vi "Read Name.vi"(8 "error in (no error)":errorcluster, 11 "bt_Send_Queue in":refnum<class "bt_Send_Queue.lvclass">) -> (0 "error out":errorcluster, 2 "Name":string, 3 "bt_Send_Queue out":refnum<class "bt_Send_Queue.lvclass">)   [LabVIEW 2021, in "BT.lvlib" / "bt_Send_Queue.lvclass"]
uses:
  bt_Send_Queue.lvclass
  bt_Send_Queue.lvclass/bt_Send_Queue.ctl
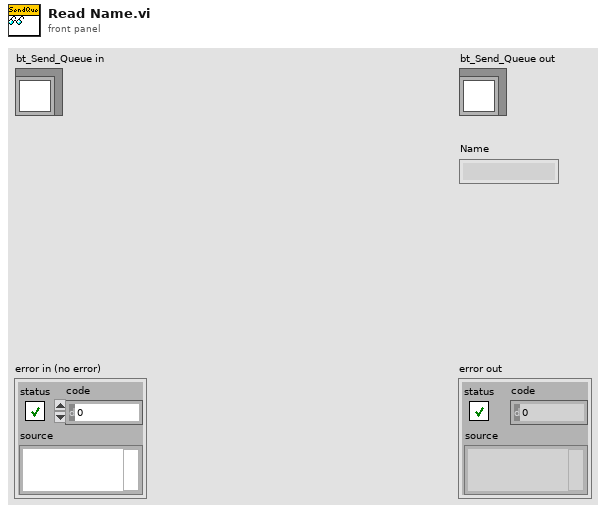
[diagram p1: front panel]
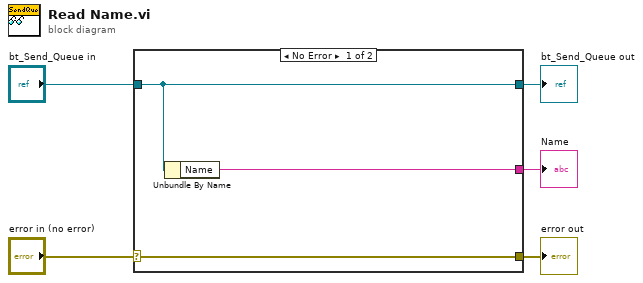
[diagram p0: block diagram]
diagram:
  n1 = case shown="No Error" "error in (no error)" {
    selector: "error in (no error)" -> [w8 w9]
    tunnel: [w8 w9] -> w4
    tunnel: [w7 w10] -> w2
    tunnel: "bt_Send_Queue in" -> [w7 w10]
    tunnel: [w6 _] -> w1
    frame No Error {
      n2 = Unbundle By Name(w7) -> ("Name"=w6:string)
    }
    frame Error {
    }
  }
  "error out" <- w4
  "bt_Send_Queue out" <- w2
  "Name" <- w1
